vi "VNA ContinuousRun.vi"(8 "error in (no error)":errorcluster, 11 "LibreVNA in":refnum<class "LibreVNA.lvclass">) -> (0 "error out":errorcluster, 3 "LibreVNA out":refnum<class "LibreVNA.lvclass">)   [LabVIEW 2023, in "LibreVNA.lvclass"]
uses:
  LibreVNA.lvclass
  LibreVNA.lvclass/LibreVNA.ctl
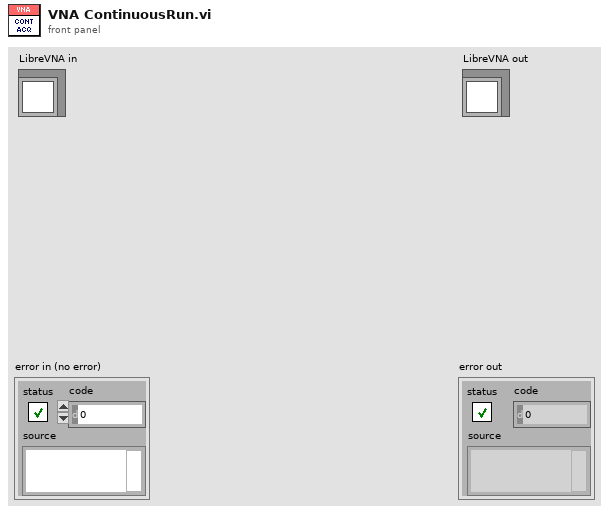
[diagram p1: front panel]
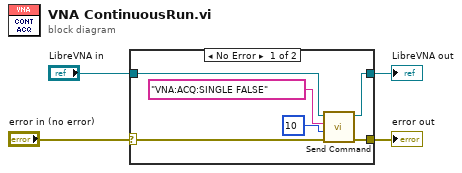
[diagram p0: block diagram]
diagram:
  n1 = case shown="No Error" "error in (no error)" {
    selector: "error in (no error)" -> [w8 w12]
    tunnel: [w7 w12] -> w3
    tunnel: [w10 w11] -> w1
    tunnel: "LibreVNA in" -> [w6 w11]
    frame No Error {
      n2 = call-dynamic "Send Command.vi"("error in (no error)"=w8, "command delay (ms)"=u32 10, "Command"="VNA:ACQ:SINGLE FALSE", "LibreVNA in"=w6) -> ("error out"=w7:errorcluster, "LibreVNA out"=w10:refnum<class "LibreVNA.lvclass">)  [unwired: 5 in, 1 out]
    }
    frame Error {
    }
  }
  "error out" <- w3
  "LibreVNA out" <- w1
